vi "Exercice Serrure.vi"() -> ()   [LabVIEW 2018]
panel:
  out "Boolean":bool
  in  "Knob 3":i64(knob) scale=0.0..9.0
  in  "Knob 2":i64(knob) scale=0.0..9.0
  in  "Knob":i64(knob) max=9 scale=0.0..9.0
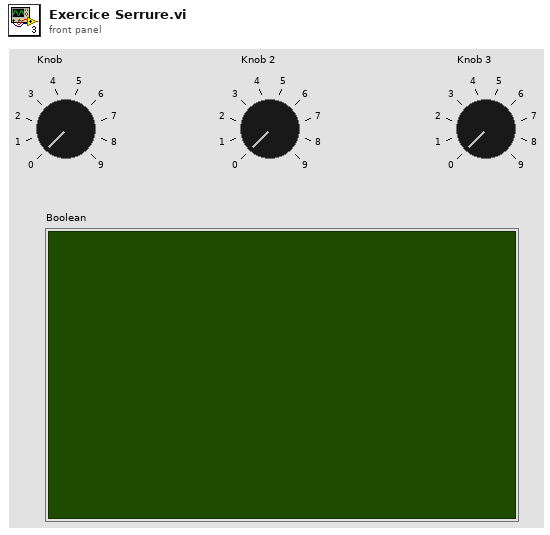
[diagram p1: front panel]
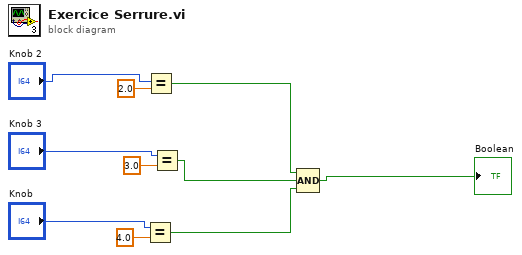
[diagram p0: block diagram]
diagram:
  n1 = Equal?(x="Knob", y=4.0) -> (x = y?=w2:bool)
  n2 = Equal?(x="Knob 2", y=2.0) -> (x = y?=w4:bool)
  n3 = Equal?(x="Knob 3", y=3.0) -> (x = y?=w3:bool)
  n4 = Compound Arithmetic op=AND(w4, w3, w2) -> (→"Boolean":bool)
